vi "Decompose LabVIEW Object - String - Library Version Value.vi"() -> ()   [LabVIEW 2017, in "Composition.Tests.lvlib"]
uses:
  Composition.Tests.lvlib
  Classes/String/String.lvclass
  Composition/Composition.lvlib
  <vilib>/addons/_JKI Toolkits/Caraya/classes/Assert/Assert.lvclass
  <vilib>/addons/_JKI Toolkits/Caraya/classes/Test/Test.lvclass
panel:
  out "error out":errorcluster
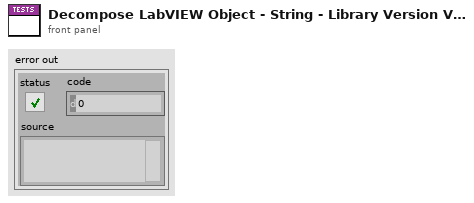
[diagram p1: front panel]
types:
  T1 = cluster{"Major":u16, "Minor":u16, "Fix":u16, "Build":u16}[]
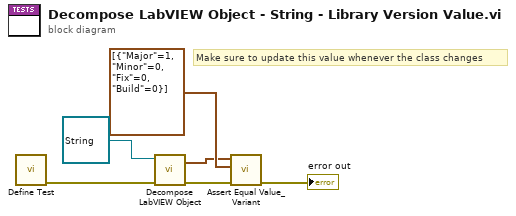
[diagram p0: block diagram]
diagram:
  # "Make sure to update this value whenever the class changes"
  n1 = call <vilib>:"Define Test.vi"() -> ("error out"=w1:errorcluster)  [unwired: 11 in]
  n2 = call "Decompose LabVIEW Object.vi"("error in (no error)"=w1, "LabVIEW Object"=refnum<class "String.lvclass"> refnum ("Reflection.Tests.lvlib:String.lvclass")) -> ("error out"=w5:errorcluster, "Library Versions"=w2:T1)  [unwired: 6 in, 2 out]
  n3 = call <vilib>:"Assert Equal Value_Variant.vi"("error in (no error)"=w5, "Y"=T1 [{"Major"=1, "Minor"=0, "Fix"=0, "Build"=0}] ("Library Versions"), "X"=w2) -> ("error out"=→"error out":errorcluster)  [unwired: 8 in]
